vi "AI_StreamingAI_MultipleChannels v9.vi"() -> ()   [LabVIEW 2013]
uses:
  <vilib>/Platform/TimedLoop/XDataNode/timing_clust.ctl
  <vilib>/Platform/TimedLoop/XDataNode/nitl_modes.ctl
  <vilib>/Platform/TimedLoop/XDataNode/wakeup.ctl
  <userlib>/DAQNavi Polymorphic VI/create/DAQNavi Create Channel(AI-Voltage).vi
  <userlib>/DAQNavi Polymorphic VI/configure/timing/DAQNavi Timing(Convert Clock).vi
  <userlib>/DAQNavi Polymorphic VI/configure/DAQNavi Get Property/AI/DAQNaviGet_AI_ConvertClock_Rate.vi
  <userlib>/DAQNavi Polymorphic VI/read/DAQNavi Read (Analog 1D Wfm NChan NSamp).vi
  <vilib>/platform/TimedLoop/XDataNode/XDataNode.xnode
  <vilib>/Platform/TimedLoop/XDataNode/XDNodeRunTimeDep.lvlib
panel:
  in  "DO":bool[](array[boolean])
  out "data":waveform(dbl)[](array[waveform])
  out "Stp Lp2":bool
  out "Stp Lp1":bool
  out "loop time":dbl format="%.6g"
  in  "Read AtoD":bool
  out "Task5":i32
  out "Test":timestamp
  out "Start":timestamp
  out "loops":bool
  out "error out":errorcluster
  out "Waveform Graph":waveform(dbl)[](graph)
  out "value range":string="+/- 5 V" caption="property value"
  out "physical channels":string="DemoDevice,BID#0/ai0:1" caption="property value"
  in  "Samples":u32=1000
  in  "samples per channel":i32=1024
  out "actual convert rate":dbl
  in  "convert clock rate":dbl=1000.0
  in  "stop":bool
  # "Please modify physical channels and value range in Channel Parameters\nthrough DAQNavi Property Assistant VI  in block diagram."
  # "Channel Parameters"
  # "Timing Parameters"
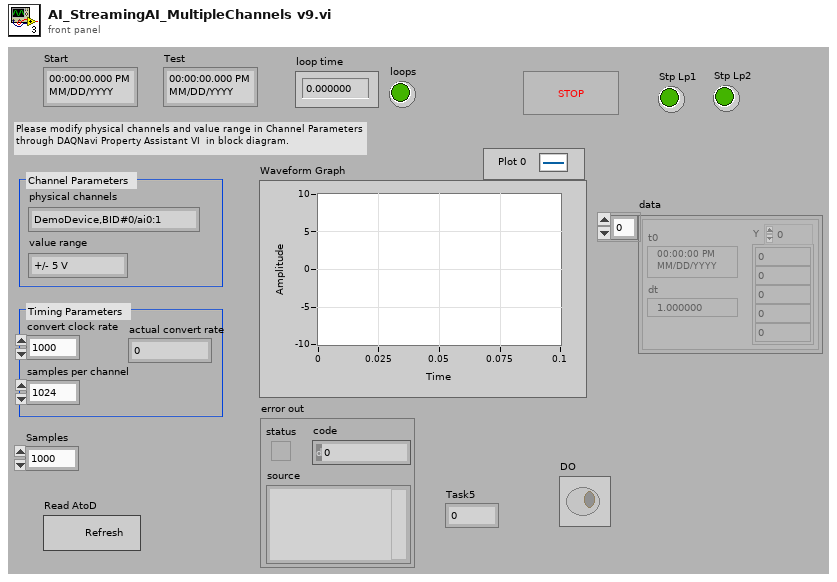
[diagram p1: front panel]
types:
  T1 = typedef "XDNodeRunTimeDep.lvlib/timing_clust.ctl" = cluster{"Expected End [f-1]":u64, "Actual End [f-1]":u64, "Finished Late? [f-1]":bool, "Expected End [i-1]":u64, "Actual End [i-1]":u64, "Finished Late? [i-1]":bool, "Expected Start [i]":u64, "Actual Start [i]":u64, "Expected Start [f]":u64, "Actual Start [f]":u64, "Source Name":string, "Structure Name":string, "Period":i64, "Deadline":i64, "Offset":i64, "Start":i64, "Priority":i32, "Timeout":i32, "Mode":T2, "Wakeup Reason":T3, "Error":errorcluster, "Source Type":string, "Secondary Source Type":string, "Global End Time":u64, "Global Start Time":u64, "Frame Duration":u64, "Iteration Duration":u64, "Assigned CPU":i32, "I/O Scan Engine Mode":u32}
  T2 = typedef "XDNodeRunTimeDep.lvlib/nitl_modes.ctl" = enum32{"No Change", "Process missed periods, maintain original phase", "Discard missed periods, maintain original phase", "Process missed periods, ignore original phase", "Discard missed periods, ignore original phase"}
  T3 = typedef "XDNodeRunTimeDep.lvlib/wakeup.ctl" = enum32{"Normal", "Aborted", "Asynchronous wakeup", "Timing source error", "Timed loop error", "Timeout"}
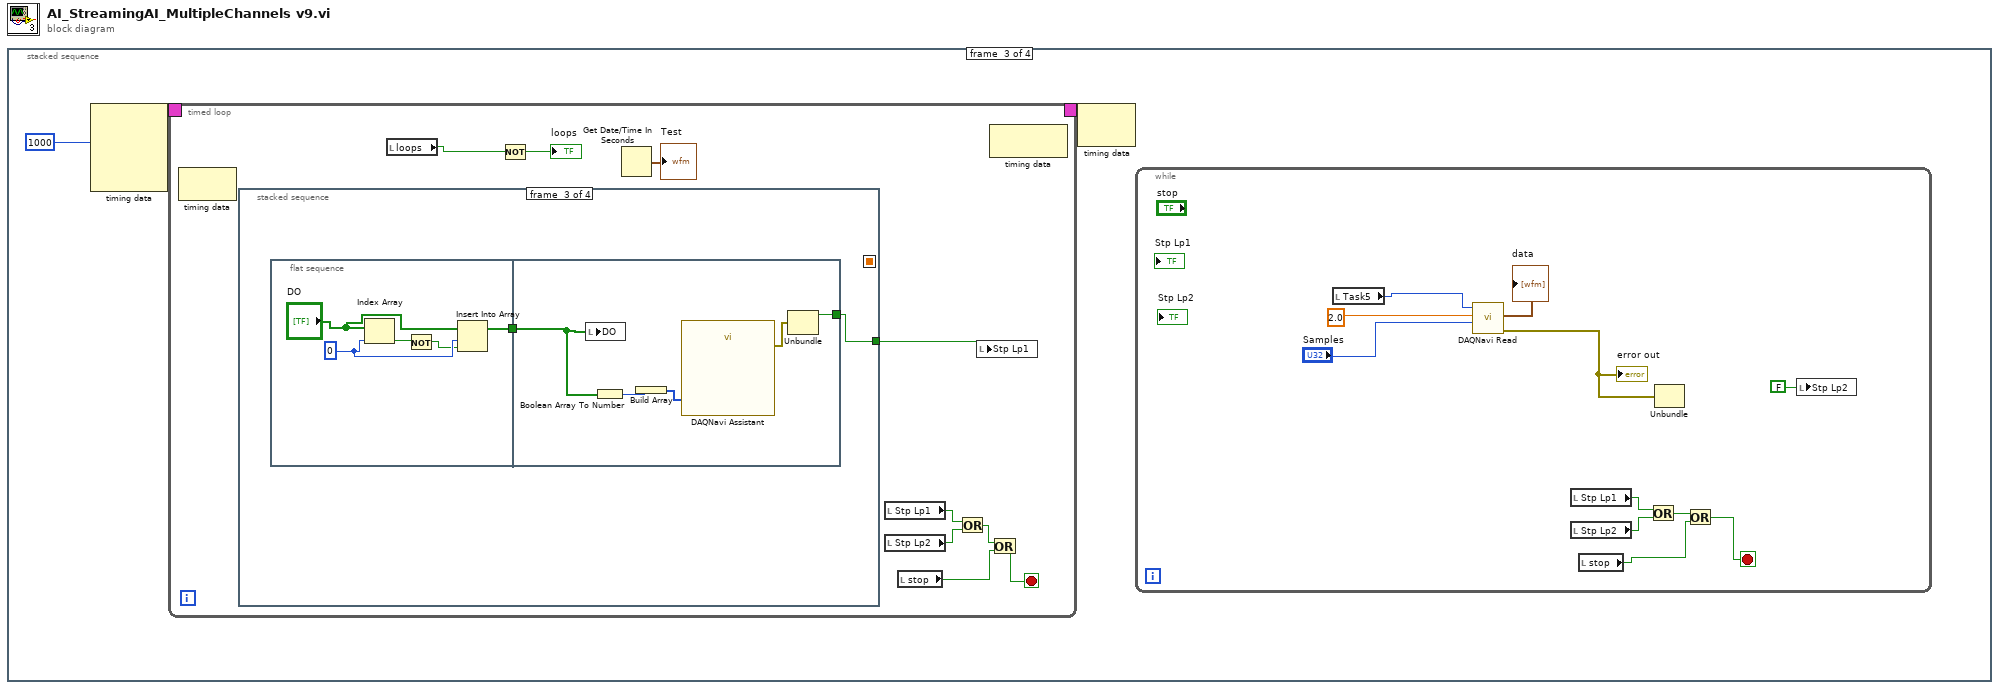
[diagram p0: block diagram]
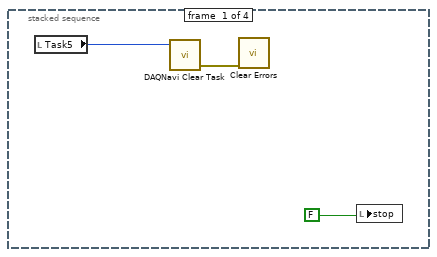
[diagram p2: hidden frame]
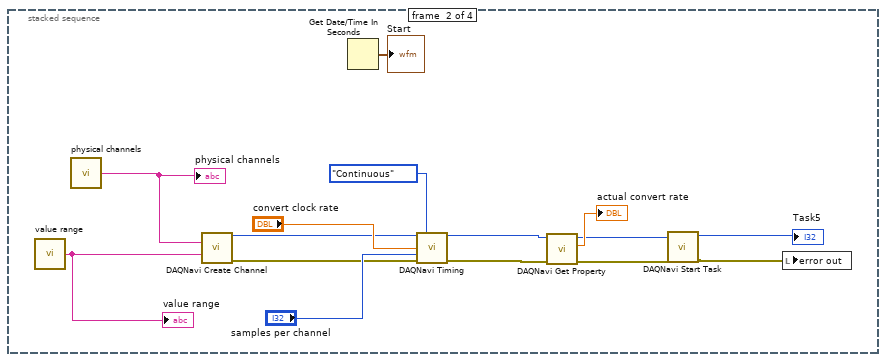
[diagram p3: hidden frame]
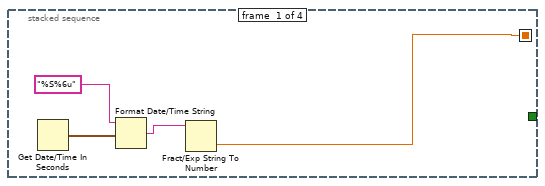
[diagram p4: hidden frame]
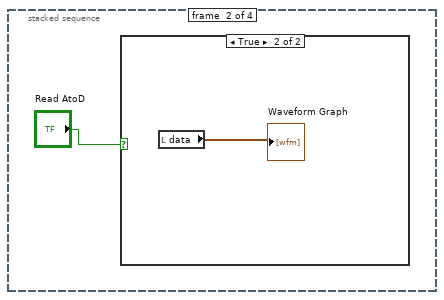
[diagram p5: hidden frame]
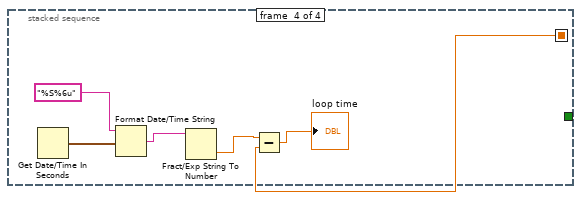
[diagram p7: hidden frame]
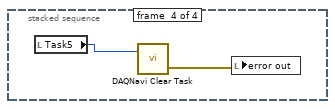
[diagram p8: hidden frame]
diagram:
  n1 = stacked-sequence {
    frame #0 {
      n2 = local read "Task5"() -> (w3:i32)
      n3 = call <userlib>:"DAQNavi Clear Task.vi"("task in"=w3) -> ("error out"=w2:errorcluster)  [unwired: 2 in]
      n4 = call <vilib>:"Clear Errors.vi"("error in (no error)"=w2) -> ()  [unwired: 6 in, 1 out]
      n5 = local write "stop"(FALSE) -> ()
    }
    frame #1 {
      n6 = call "value range"() -> ("property value"=w17:string)  [unwired: 1 out]
      "value range" <- w17
      n7 = call "physical channels"() -> ("property value"=w16:string)  [unwired: 1 out]
      "physical channels" <- w16
      n8 = call-poly <userlib>:"DAQNavi Create Channel.vi"("physical channels"=w16, "value range"=w17) -> ("task out"=w8:i32, "error out"=w9:errorcluster)  [unwired: 3 in, 9 out]
      n9 = Get Date/Time In Seconds() -> (seconds since 1Jan1904=→"Start":timestamp)
      n10 = call-poly <userlib>:"DAQNavi Timing.vi"("task in"=w8, "sample mode"=enum16{"Finite", "Continuous"}."Continuous", "rate"="convert clock rate", "samples per channel"="samples per channel", "error in (no error)"=w9) -> ("task out"=w12:i32, "error out"=w13:errorcluster)  [unwired: 1 in, 8 out]
      n11 = call-poly <userlib>:"DAQNavi Get Property.vi"("error in (no error)"=w13, "task in"=w12) -> ("error out"=w6:errorcluster, "rate"=→"actual convert rate":dbl, "task out"=w7:i32)  [unwired: 7 out]
      n12 = call <userlib>:"DAQNavi Start Task.vi"("error in (no error)"=w6, "task in"=w7) -> ("error out"=w5:errorcluster, "task out"=→"Task5":i32)  [unwired: 8 in]
      n13 = local write "error out"(w5) -> ()
    }
    frame #2 {
      n14 = node-c288(1000) -> (w21:T1)  [unwired: 3 in]
      n15 = timed-loop {
        timing: w21 -> [_]
        timing-out: [_] -> w20
        stop <- w33 stop-if-true
        n16 = node-c288() -> ()  [unwired: 1 in, 1 out]
        n17 = stacked-sequence {
          seq-local: [w42 _ _ _] -> [_ _ _ w60]
          tunnel: [_ _ w48 _] -> w38
          frame #0 {
            n18 = Get Date/Time In Seconds() -> (seconds since 1Jan1904=w44:timestamp)
            n19 = Format Date/Time String(time format string (%c)="%S%6u", seconds (now)=w44) -> (date/time string=w43:string)  [unwired: 1 in]
            n20 = Fract/Exp String To Number(string=w43) -> (number=w42:dbl)  [unwired: 3 in, 1 out]
          }
          frame #1 {
            n21 = case shown="True" "Read AtoD" {
              frame False {
              }
              frame True {
                n22 = local read "data"() -> (→"Waveform Graph":waveform(dbl)[])
              }
            }
          }
          frame #2 {
            n23 = flat-sequence {
              tunnel: [w50] -> w49
              tunnel: w49 -> [w58]
              tunnel: [w57] -> w48
              frame #0 {
                w54 = 0
                n24 = Index Array(array="DO", index=w54) -> (element=w52:bool)
                n25 = Not(x=w52) -> (.not. x?=w53:bool)
                n26 = Insert Into Array(array="DO", index=w54, new element=w53) -> (w50:bool[])
              }
              frame #1 {
                n27 = local write "DO"(w58) -> ()
                n28 = Boolean Array To Number(Boolean array=w58) -> (number=w59:u32)
                n29 = Build Array(w59) -> (w56:u32[])
                n30 = call "DAQNavi Assistant"("dataIn(U8Array)"=w56) -> ("error out"=w55:errorcluster)  [unwired: 26 in]
                n31 = Unbundle(w55) -> ("status"=w57:bool)  [unwired: 2 out]
              }
            }
          }
          frame #3 {
            n32 = Get Date/Time In Seconds() -> (seconds since 1Jan1904=w64:timestamp)
            n33 = Format Date/Time String(time format string (%c)="%S%6u", seconds (now)=w64) -> (date/time string=w63:string)  [unwired: 1 in]
            n34 = Fract/Exp String To Number(string=w63) -> (number=w62:dbl)  [unwired: 3 in, 1 out]
            n35 = Subtract(x=w62, y=w60) -> (x-y=→"loop time":dbl)
          }
        }
        n36 = local read "loops"() -> (w40:bool)
        n37 = Not(x=w40) -> (.not. x?=→"loops":bool)
        n38 = Get Date/Time In Seconds() -> (seconds since 1Jan1904=→"Test":timestamp)
        n39 = local read "Stp Lp1"() -> (w37:bool)
        n40 = local read "Stp Lp2"() -> (w36:bool)
        n41 = local read "stop"() -> (w34:bool)
        n42 = Or(x=w37, y=w36) -> (x .or. y?=w35:bool)
        n43 = local write "Stp Lp1"(w38) -> ()
        n44 = node-c288() -> ()  [unwired: 1 in, 1 out]
        n45 = Or(x=w35, y=w34) -> (x .or. y?=w33:bool)
      }
      n46 = node-c288(w20) -> ()  [unwired: 1 out]
      n47 = while {
        stop <- w28 stop-if-true
        n48 = local read "Task5"() -> (w26:i32)
        n49 = call-poly <userlib>:"DAQNavi Read.vi"("number of samples per channel to read"="Samples", "timeout"=2.0, "task in"=w26) -> ("error out"=w23:errorcluster, "data"=→"data":waveform(dbl)[])  [unwired: 6 in, 1 out]
        "error out" <- w23
        n50 = local read "Stp Lp1"() -> (w32:bool)
        n51 = local read "Stp Lp2"() -> (w31:bool)
        n52 = local read "stop"() -> (w29:bool)
        n53 = Or(x=w32, y=w31) -> (x .or. y?=w30:bool)
        n54 = Unbundle(w23) -> ()  [unwired: 3 out]
        n55 = Or(x=w30, y=w29) -> (x .or. y?=w28:bool)
        n56 = local write "Stp Lp2"(FALSE) -> ()
      }
    }
    frame #3 {
      n57 = local read "Task5"() -> (w72:i32)
      n58 = call <userlib>:"DAQNavi Clear Task.vi"("task in"=w72) -> ("error out"=w73:errorcluster)  [unwired: 1 in, 1 out]
      n59 = local write "error out"(w73) -> ()
    }
  }
